vi "PS_check_ramping_done.vi"(2 "Magnet PS":u16(ring) items=["Resistive Magnet", "SCM2", "SCM1", "Generic SC power supply", "PPMS"]) -> (0 "PS status":T1(ring))   [LabVIEW 2020]
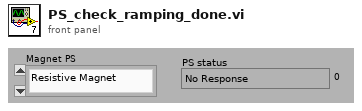
[diagram p1: front panel]
types:
  T1 = enum16{"No Response", "Ramping to programmed field ", "Holding at programmed field", "Paused", "Ramp Manual Up", "Ramp Manual Down", "Ramping to Zero", "QUENCH", "Heating Persistence Switch", "At Zero Current"}
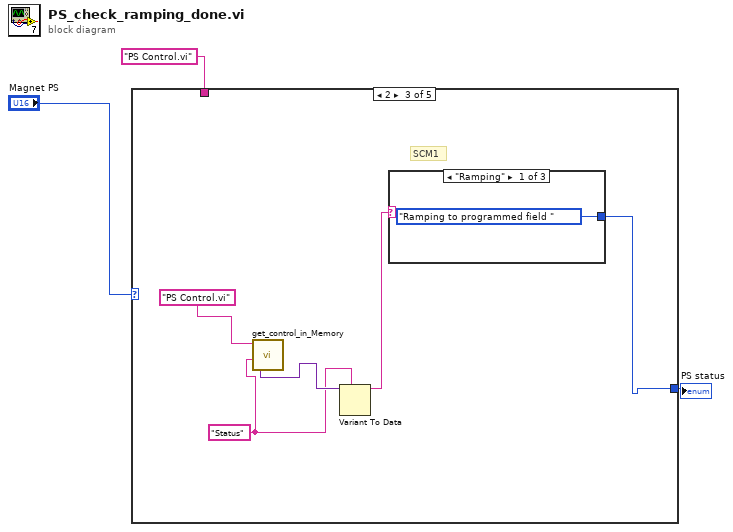
[diagram p0: block diagram]
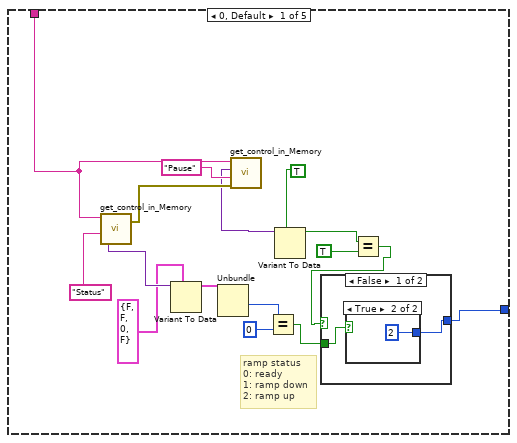
[diagram p2: hidden frame]
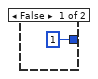
[diagram p3: hidden frame]
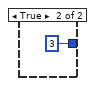
[diagram p4: hidden frame]
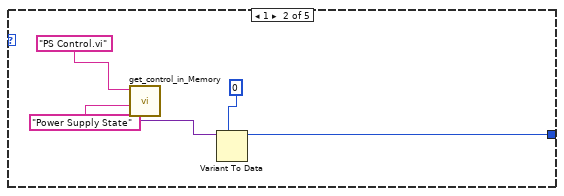
[diagram p5: hidden frame]
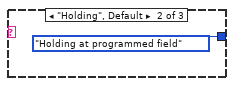
[diagram p6: hidden frame]
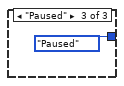
[diagram p7: hidden frame]
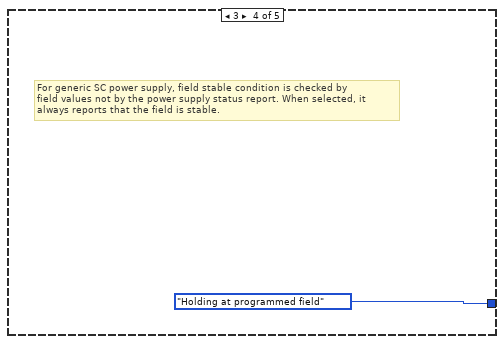
[diagram p8: hidden frame]
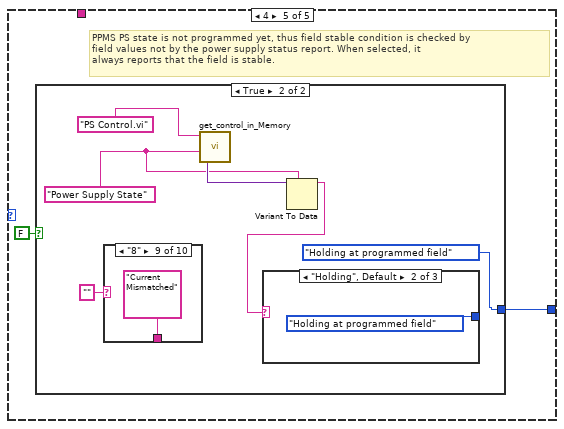
[diagram p9: hidden frame]
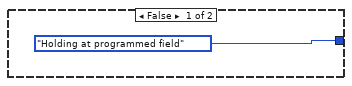
[diagram p10: hidden frame]
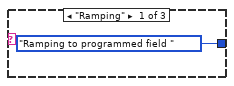
[diagram p11: hidden frame]
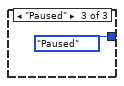
[diagram p12: hidden frame]
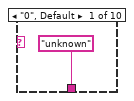
[diagram p13: hidden frame]
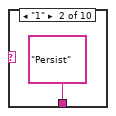
[diagram p14: hidden frame]
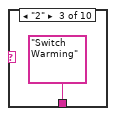
[diagram p15: hidden frame]
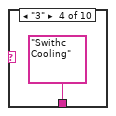
[diagram p16: hidden frame]
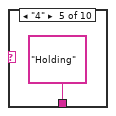
[diagram p17: hidden frame]
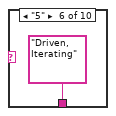
[diagram p18: hidden frame]
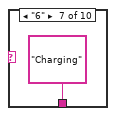
[diagram p19: hidden frame]
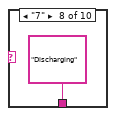
[diagram p20: hidden frame]
diagram:
  n1 = case shown="2" "Magnet PS" {
    tunnel: "PS Control.vi" ("VI Name") -> [w12 _ _ _ _]
    tunnel: [w15 w25 w31 T1."Holding at programmed field" ("PS status") w39] -> w1
    frame 0, Default {
      # "ramp status\n0: ready\n1: ramp down\n2: ramp up"
      n2 = call "get_control_in_Memory.vi"("Control Name"="Status", "VI Name"=w12) -> ("error out 2"=w13:errorcluster, "Value"=w18:variant)  [unwired: 2 in]
      n3 = Variant To Data(type=cluster{bool, bool, "Ramp Status":u16, bool} {FALSE, FALSE, "Ramp Status"=0, FALSE} ("Status"), Variant=w18) -> (data=w16:cluster{bool, bool, "Ramp Status":u16, bool})  [unwired: 1 in, 1 out]
      n4 = Unbundle(w16) -> ("Ramp Status"=w5:u16)  [unwired: 3 out]
      n5 = call "get_control_in_Memory.vi"("error in (no error)"=w13, "Control Name"="Pause", "VI Name"=w12) -> ("Value"=w11:variant)  [unwired: 1 in, 1 out]
      n6 = Equal?(x=w5, y=u16 0) -> (x = y?=w6:bool)
      n7 = Variant To Data(type=TRUE ("y"), Variant=w11) -> (data=w8:bool)  [unwired: 1 in, 1 out]
      n8 = Equal?(x=w8, y=TRUE) -> (x = y?=w7:bool)
      n9 = case shown="False" w7 {
        tunnel: [w20 3] -> w15
        tunnel: w6 -> [w21 _]
        frame False {
          n10 = case shown="True" w21 {
            tunnel: [1 2] -> w20
            frame False {
            }
            frame True {
            }
          }
        }
        frame True {
        }
      }
    }
    frame 1 {
      n11 = call "get_control_in_Memory.vi"("Control Name"="Power Supply State", "VI Name"="PS Control.vi") -> ("Value"=w27:variant)  [unwired: 2 in, 1 out]
      n12 = Variant To Data(type=0, Variant=w27) -> (data=w25:i32)  [unwired: 1 in, 1 out]
    }
    frame 2 {
      w30 = "Status" ("Control Name")
      # "SCM1"
      n13 = call "get_control_in_Memory.vi"("Control Name"=w30, "VI Name"="PS Control.vi") -> ("Value"=w33:variant)  [unwired: 2 in, 1 out]
      n14 = Variant To Data(type=w30, Variant=w33) -> (data=w32:string)  [unwired: 1 in, 1 out]
      n15 = case shown="\"Ramping\"" w32 {
        tunnel: [T1."Ramping to programmed field " ("PS status") T1."Holding at programmed field" ("PS status") T1."Paused" ("PS status")] -> w31
        frame "Ramping" {
        }
        frame "Holding", Default {
        }
        frame "Paused" {
        }
      }
    }
    frame 3 {
      # "For generic SC power supply, field stable condition is checked by\nfield values not by the power supply status report. When selected, it \nalways reports that the field is stable."
    }
    frame 4 {
      # "PPMS PS state is not programmed yet, thus field stable condition is checked by\nfield values not by the power supply status report. When selected, it \nalways reports that the field is stable."
      n16 = case shown="True" FALSE {
        tunnel: [T1."Holding at programmed field" ("PS status") T1."Holding at programmed field" ("PS status")] -> w39
        frame False {
        }
        frame True {
          w45 = "Power Supply State" ("Control Name")
          n17 = case shown="\"8\"" "" {
            tunnel: ["unknown" "Persist" "Switch Warming" "Swithc Cooling" "Holding" "Driven, Iterating" "Charging" "Discharging" "Current Mismatched" "Total Failure"] -> _
            frame "0", Default {
            }
            frame "1" {
            }
            frame "2" {
            }
            frame "3" {
            }
            frame "4" {
            }
            frame "5" {
            }
            frame "6" {
            }
            frame "7" {
            }
            frame "8" {
            }
            frame "15" {
            }
          }
          n18 = call "get_control_in_Memory.vi"("Control Name"=w45, "VI Name"="PS Control.vi") -> ("Value"=w46:variant)  [unwired: 2 in, 1 out]
          n19 = Variant To Data(type=w45, Variant=w46) -> (data=w44:string)  [unwired: 1 in, 1 out]
          n20 = case shown="\"Holding\", Default" w44 {
            tunnel: [T1."Ramping to programmed field " ("PS status") T1."Holding at programmed field" ("PS status") T1."Paused" ("PS status")] -> _
            frame "Ramping" {
            }
            frame "Holding", Default {
            }
            frame "Paused" {
            }
          }
        }
      }
    }
  }
  "PS status" <- w1
